vi "(SubVI)_ReadPolyFitCoeffs_convert_WtoV.vi"(4 "Optical Power (mW)":dbl, 5 "file path (use dialog)":path=path "C:/Users/Alana/Documents/Rex-Dropbox/Dropbox/BIST lab/1-Projects/ClosedLoop/testing_results/StimPowerMeasurement/mWtoV.bin") -> (0 "error out":errorcluster, 2 "Voltage (V)":dbl)   [LabVIEW 2012]
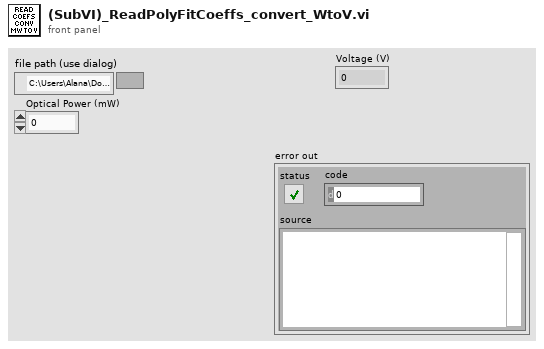
[diagram p1: front panel]
types:
  T1 = enum16{"big-endian, network order", "native, host order", "little-endian"}
  T2 = enum16{"open", "replace", "create", "open or create", "replace or create", "replace or create with confirmation"}
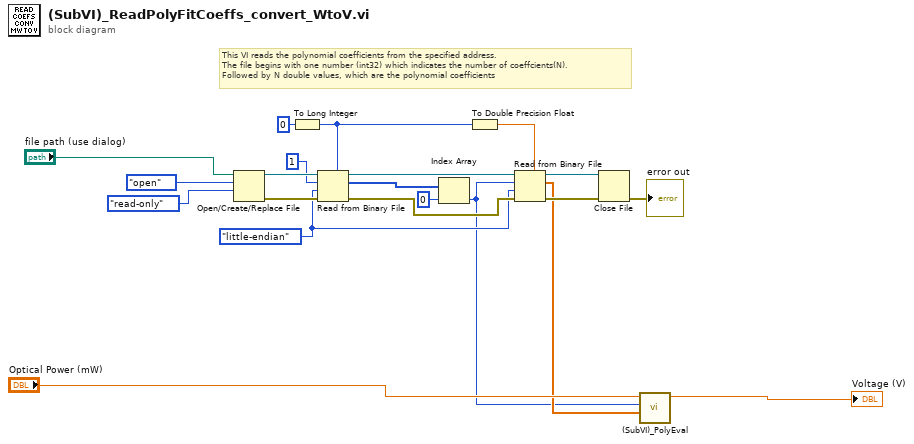
[diagram p0: block diagram]
diagram:
  w10 = T1."little-endian" ("byte order (0:big-endian, network order)")
  # "This VI reads the polynomial coefficients from the specified address.\nThe file begins with one number (int32) which indicates the number of coeffcients(N).\nFollowed by N double values, which are the polynomial coefficients"
  n1 = Open/Create/Replace File(file path (use dialog)="file path (use dialog)", operation (0:open)=T2."open", access (0:read/write)=enum16{"read/write", "read-only", "write-only"}."read-only") -> (refnum out=w18:refnum<file>, error out=w13:errorcluster)  [unwired: 3 in, 1 out]
  n2 = To Long Integer(number=0) -> (32bit integer=w6:i32)
  n3 = Read from Binary File(5:w6, 8:w13, 9:w10, 10:1 ("count (1)"), 11:w18) -> (0:w12:errorcluster, 2:w15:i32[], 3:w16:refnum<file>)  [unwired: 1 in, 1 out]
  n4 = Index Array(array=w15, index=0) -> (element=w1:i32)
  n5 = To Double Precision Float(number=w6) -> (double precision float=w5:dbl)
  n6 = Read from Binary File(5:w5, 8:w12, 9:w10, 10:w1, 11:w16) -> (0:w8:errorcluster, 2:w2:dbl[], 3:w9:refnum<file>)  [unwired: 1 in, 1 out]
  n7 = Close File(refnum=w9, error in=w8) -> (error out=→"error out":errorcluster)  [unwired: 1 out]
  n8 = call "(SubVI)_PolyEval.vi"("Poly Coefficients"=w2, "No Of Coeffs"=w1, "Optical Power (mW)"="Optical Power (mW)") -> ("Voltage (V)"=→"Voltage (V)":dbl)  [unwired: 8 in]
